vi "MaskImage_Red.vi"(2 "Mask in":T1 {"Dialogs" format="%.0b"}, 3 "Image":T1 {"Dialogs" format="%.0b"}) -> (1 "Image Out":T1 {"Dialogs" format="%.0b"})   [LabVIEW 2010]
doc: "This vi will mask an image. It will mask all planes or each individual color plane of a color image depending on which poly selection is chosen."
uses:
  <userlib>/ImageProcessing/QTLIB_2595_LV86/QT_Image.ctl
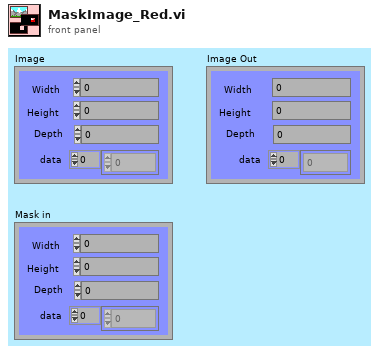
[diagram p1: front panel]
types:
  T1 = typedef "QT_Image.ctl" = cluster{"Width":i32, "Height":i32, "Depth":i32, "data":u8[], "Compressed data":u8[], "Color table":u32[], "Duration":i32, "Options":i32, "Timestamp":i32, "ID":i32, "Reserved":i32, "Dialogs":u32}
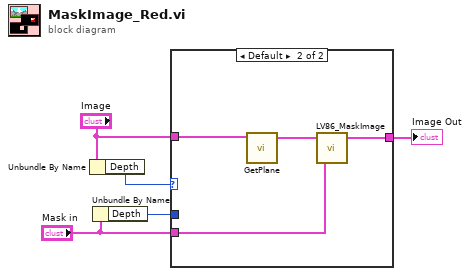
[diagram p0: block diagram]
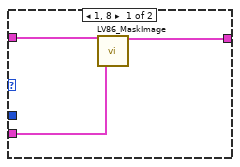
[diagram p2: hidden frame]
diagram:
  n1 = Unbundle By Name("Image") -> ("Depth"=w3:i32)
  n2 = Unbundle By Name("Mask in") -> ("Depth"=w1:i32)
  n3 = case shown="Default" w3 {
    tunnel: "Mask in" -> [w7 w10]
    tunnel: [w6 w9] -> w5
    tunnel: "Image" -> [w8 w12]
    tunnel: w1 -> [_ _]
    frame 1, 8 {
      n4 = call <userlib>:"LV86_MaskImage.vi"("Mask in"=w7, "Image"=w8) -> ("Image Out"=w6:T1)  [unwired: 1 in]
    }
    frame Default {
      n5 = call <userlib>:"GetPlane.vi"("Image In"=w12) -> ("Red Plane Out"=w11:T1)  [unwired: 2 out]
      n6 = call <userlib>:"LV86_MaskImage.vi"("Mask in"=w10, "Image"=w11) -> ("Image Out"=w9:T1)  [unwired: 1 in]
    }
  }
  "Image Out" <- w5
